vi "VISA_clear.vi"   [LabVIEW 2023]
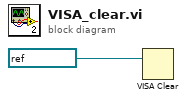
[diagram p0: block diagram]
diagram:
  n1 = VISA Clear(VISA resource name=refnum<visa-resource-name> "COM17") -> ()  [unwired: 1 in, 2 out]
